vi "Set Terminal Mode.vi"(8 "error in (no error)":errorcluster, 10 "Terminal Mode":T1, 11 "Value Editor Base in":refnum<class "Value Editor Base.lvclass">) -> (0 "error out":errorcluster, 3 "Value Editor Base out":refnum<class "Value Editor Base.lvclass">)   [LabVIEW 2020, in "Value Editor Base.lvclass"]
uses:
  Value Editor Base.lvclass
  Terminal Mode.ctl
  Terminal Mode Data.ctl
  Value Editor Base.lvclass/Value Editor Base.ctl
  FlexBlocks.lvlib
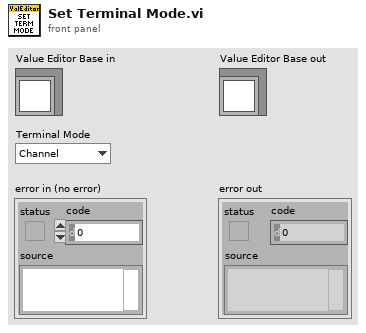
[diagram p1: front panel]
types:
  T1 = typedef "FlexBlocks.lvlib/Terminal Mode.ctl" = enum16{"Channel", "Config", "Value", "Control Ref"}
  T2 = typedef "Value Editor Base.lvclass/Terminal Mode Data.ctl" = cluster{"Terminal Mode":T1}
  T3 = typedef "Value Editor Base.lvclass/Ref Data.ctl" = cluster{"Type Descriptor":T4, "Terminal Mode":T1, "Value":variant}
  T4 = typedef "FlexBlocks.lvlib/Type Descriptor.ctl" = cluster{"Name":string, "Direction":T5, "Default":variant, "Min":variant, "Max":variant, "Step":variant, "Value Mode":T6, "Required":bool, "Connpane Index":i32, "Special Terminal":T7, "Color":u32, "Options":string[], "Type String":string, "Sort":i32, "Item Path":path}
  T5 = typedef "FlexBlocks.lvlib/Terminal Direction.ctl" = enum16{"Sink", "Source"}
  T6 = typedef "FlexBlocks.lvlib/Value Mode.ctl" = enum16{"Normal", "Range", "Select"}
  T7 = typedef "FlexBlocks.lvlib/Special Terminal.ctl" = enum16{"None", "Action", "Init", "Tag", "State in", "State out", "Error"}
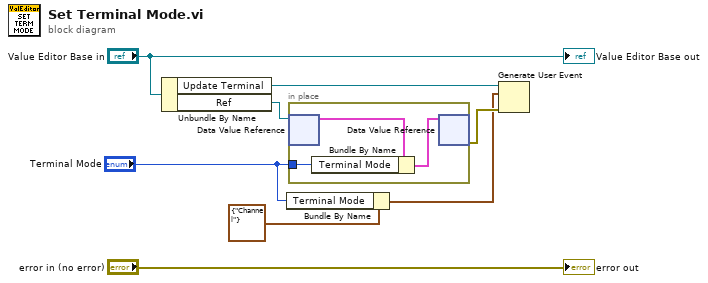
[diagram p0: block diagram]
diagram:
  n1 = Unbundle By Name("Value Editor Base in") -> ("Update Terminal"=w5:refnum<user-event>, "Ref"=w7:refnum<data-value>)
  n2 = Bundle By Name(cluster=T2 {"Terminal Mode"=enum."Channel"} ("Terminal Mode Data"), "Terminal Mode"="Terminal Mode") -> (w1:T2)
  n3 = in-place {
    in-place-border: "Terminal Mode" -> [w9]
    n4 = in-place-dvr #1(w7) -> (w11:T3)  [unwired: 1 out]
    n5 = Bundle By Name(cluster=w11, "Terminal Mode"=w9) -> (w10:T3)
    n6 = in-place-dvr #1(w10) -> (w4:errorcluster)  [unwired: 1 out]
  }
  n7 = Generate User Event(user event=w5, event data cluster=w1, error in=w4) -> ()  [unwired: 1 in, 2 out]
  "error out" <- "error in (no error)"
  "Value Editor Base out" <- "Value Editor Base in"
